vi "Format Control Data Element.vi"(6 "Unsupported Error":errorcluster, 8 "error in (no error)":errorcluster, 10 "Content Type in":string, 11 "Data":variant) -> (0 "error out":errorcluster, 2 "Content Type out":string, 3 "JSON string":string)   [LabVIEW 2023, in "Response.lvclass"]
uses:
  Response.lvclass
  <vilib>/Utility/Data Type/Type Definitions/Data Type.ctl
  Helpers/UTC.ctl
  <vilib>/Utility/Data Type/NI_Data Type.lvlib
  <vilib>/wsapi/NI_WebServices.lvlib
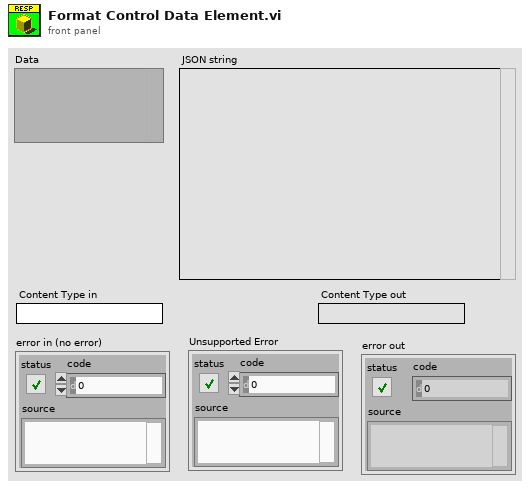
[diagram p1: front panel]
types:
  T1 = typedef "NI_Data Type.lvlib/Data Type.ctl" = enum8{"Invalid Type", "Void", "I8", "I16", "I32", "I64", "U8", "U16", "U32", "U64", "Single Float", "Double Float", "Extended Float", "Single Complex", "Double Complex", "Extended Complex", "Enum U8", "Enum U16", "Enum U32", "Enum U64", "Single Float With Unit", "Double Float With Unit", "Extended Float With Unit", "Single Complex with Unit", "Double Complex with Unit", "Extended Complex with Unit", "Boolean", "String", "Path", "Picture", "Tag", "Array", "Cluster", "Variant", "LV Variant", "Waveform", "Timestamp", "Digital Waveform", "Digital Data", "ExpressData", "Refnum", "External Data", "VI", "Poly VI", "LabVIEW Class Instance", "Fixed Point", "Set Collection", "Map Collection"}
  T2 = typedef "NI_Data Type.lvlib/Type Definition Info.ctl" = cluster{"Name":string, "Timestamp":u32}
  T3 = typedef "UTC.ctl" = string
  T4 = cluster{"t0":timestamp, "Y":dbl[], "dt":dbl, "attributes":variant}
  T5 = cluster{"t0":timestamp, "dt":dbl, "attributes":variant, "Y":digitaldata}
  T6 = typedef "imagedata.ctl" = cluster{"image type":i32, "image depth":i32, "image":u8[], "mask":u8[], "colors":u32[], "Rectangle":cluster{"left":i16, "top":i16, "right":i16, "bottom":i16}}
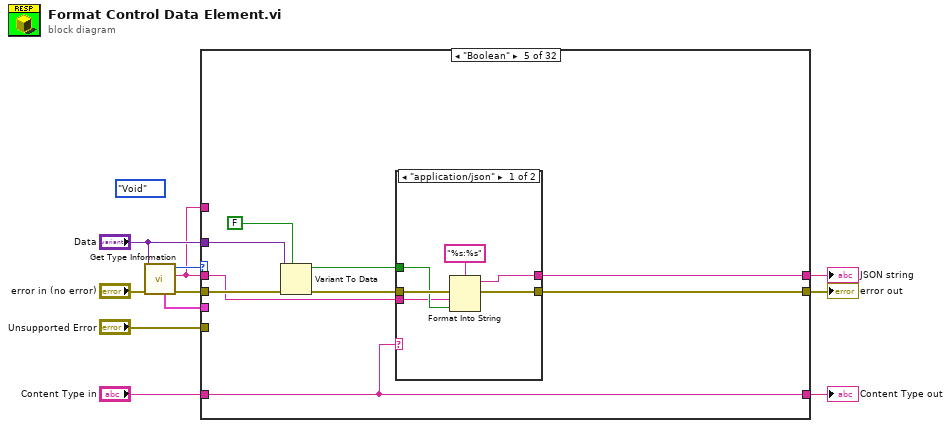
[diagram p0: block diagram]
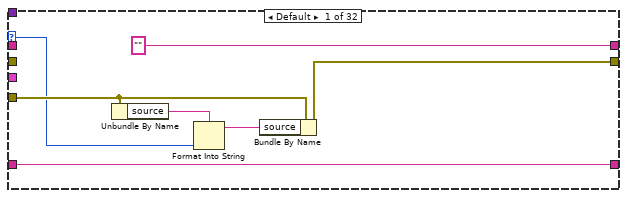
[diagram p2: hidden frame]
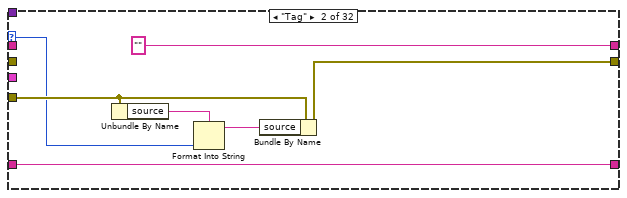
[diagram p3: hidden frame]
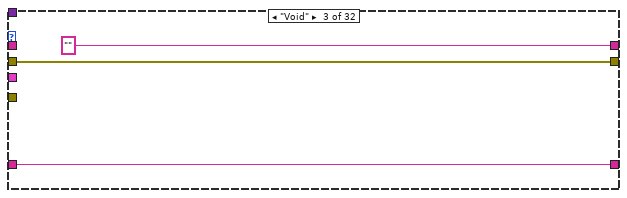
[diagram p4: hidden frame]
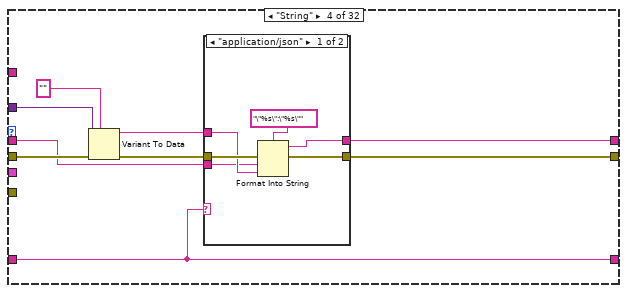
[diagram p5: hidden frame]
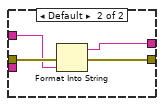
[diagram p6: hidden frame]
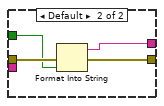
[diagram p7: hidden frame]
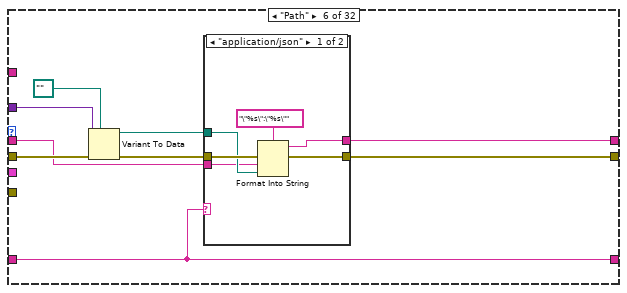
[diagram p8: hidden frame]
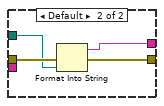
[diagram p9: hidden frame]
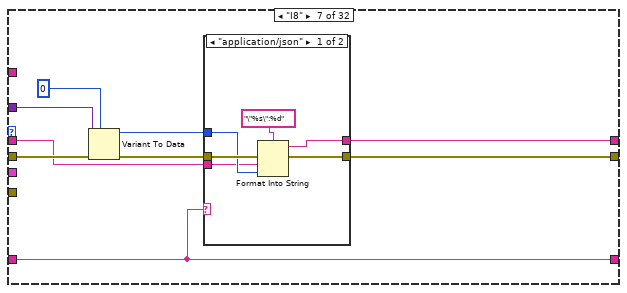
[diagram p10: hidden frame]
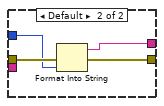
[diagram p11: hidden frame]
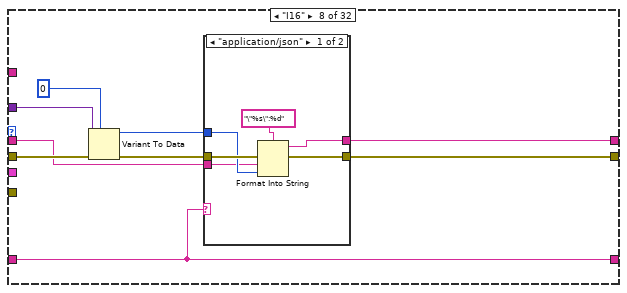
[diagram p12: hidden frame]
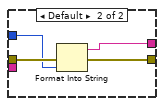
[diagram p13: hidden frame]
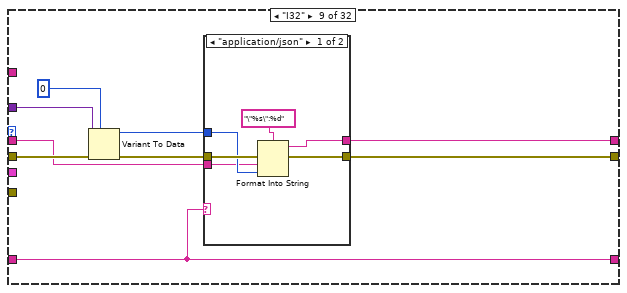
[diagram p14: hidden frame]
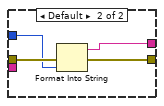
[diagram p15: hidden frame]
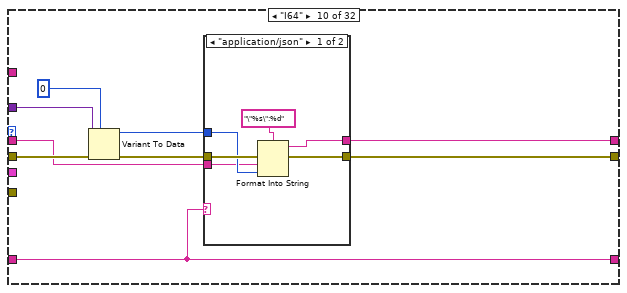
[diagram p16: hidden frame]
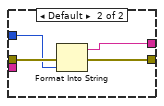
[diagram p17: hidden frame]
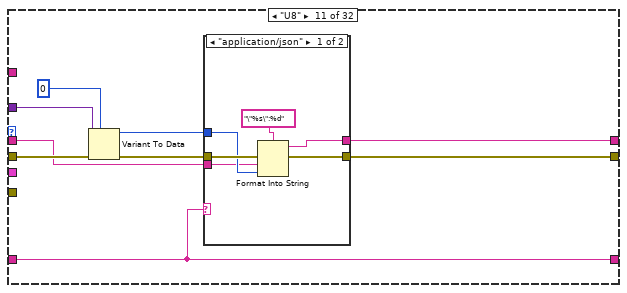
[diagram p18: hidden frame]
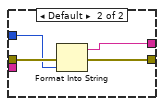
[diagram p19: hidden frame]
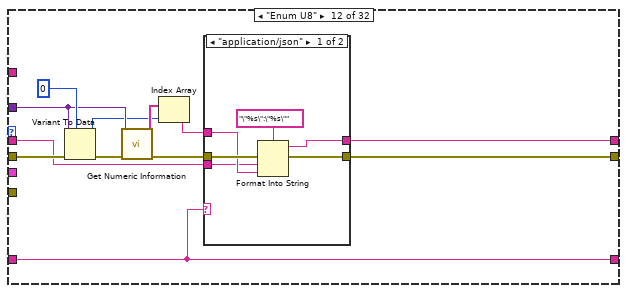
[diagram p20: hidden frame]
diagram:
  (unwired) Data_Type."Void" ("type")
  n1 = call <vilib>:"Get Type Information.vi"("error in (no error)"="error in (no error)", "variant"="Data") -> ("error out"=w7:errorcluster, "name"=w1:string, "type"=w8:T1, "type definition info"=w9:T2)  [unwired: 5 in, 1 out]
  n2 = case shown="\"Boolean\"" w8 {
    selector: w8 -> [w12 w19 _ _ _ _ _ _ _ _ _ _ _ _ _ _ _ _ _ _ _ _ _ _ _ _ _ _ _ _ _ _]
    tunnel: w7 -> [_ _ w28 w37 w56 w75 w94 w113 w132 w151 w170 w192 w214 w236 w258 w277 w296 w315 w334 w353 w372 w391 w410 w429 w449 w478 w494 w505 w514 w528 w1329 w1344]
    tunnel: w9 -> [_ _ _ _ _ _ _ _ _ _ _ _ _ _ _ _ _ _ _ _ _ _ _ _ _ _ _ _ _ _ _ _]
    tunnel: [w15 w22 w28 w34 w53 w72 w91 w110 w129 w148 w167 w191 w213 w235 w257 w274 w293 w312 w331 w350 w369 w388 w407 w426 w446 w474 w491 w502 w508 w530 w1320 w1352] -> w4
    tunnel: ["" "" "" w32 w51 w70 w89 w108 w127 w146 w165 w190 w212 w234 w256 w272 w291 w310 w329 w348 w367 w386 w405 w424 w444 w470 w487 w498 w506 w519 w1319 w1351] -> w3
    tunnel: "Data" -> [_ _ _ w36 w55 w74 w93 w112 w131 w150 w169 w185 w207 w229 w251 w276 w295 w314 w333 w352 w371 w390 w409 w428 w448 w477 w493 w504 w513 w527 w1328 w1346]
    tunnel: "Content Type in" -> [w18 w25 w26 w30 w49 w68 w87 w106 w125 w144 w163 w188 w210 w232 w254 w270 w289 w308 w327 w346 w365 w384 w403 w422 w442 w471 w488 w499 _ _ _ _]
    tunnel: [w18 w25 w26 w30 w49 w68 w87 w106 w125 w144 w163 w188 w210 w232 w254 w270 w289 w308 w327 w346 w365 w384 w403 w422 w442 w472 w489 w500 "image/png" "application/json" w1318 w1350] -> w2
    tunnel: "Unsupported Error" -> [w16 w23 _ _ _ _ _ _ _ _ _ _ _ _ _ _ _ _ _ _ _ _ _ _ _ w473 w490 w501 _ w521 w1325 w1357]
    tunnel: w1 -> [_ _ _ w29 w48 w67 w86 w105 w124 w143 w162 w187 w209 w231 w253 w269 w288 w307 w326 w345 w364 w383 w402 w421 w441 _ _ _ _ _ _ _]
    tunnel: w1 -> [_ _ _ _ _ _ _ _ _ _ _ _ _ _ _ _ _ _ _ _ _ _ _ _ _ _ _ _ _ w516 w1315 _]
    frame Default {
      n3 = Unbundle By Name(w16) -> ("source"=w14:string)
      n4 = Format Into String(format string=w14, w12) -> (resulting string=w13:string)  [unwired: 2 in, 1 out]
      n5 = Bundle By Name(cluster=w16, "source"=w13) -> (w15:errorcluster)
    }
    frame "Tag" {
      n6 = Unbundle By Name(w23) -> ("source"=w21:string)
      n7 = Format Into String(format string=w21, w19) -> (resulting string=w20:string)  [unwired: 2 in, 1 out]
      n8 = Bundle By Name(cluster=w23, "source"=w20) -> (w22:errorcluster)
    }
    frame "Void" {
    }
    frame "String" {
      n9 = Variant To Data(error in=w37, type="", Variant=w36) -> (data=w33:string, error out=w35:errorcluster)
      n10 = case shown="\"application/json\"" w30 {
        tunnel: w35 -> [w43 w47]
        tunnel: [w42 w46] -> w34
        tunnel: w33 -> [w39 w45]
        tunnel: [w40 w44] -> w32
        tunnel: w29 -> [w38 _]
        frame "application/json" {
          n11 = Format Into String(format string="\"%s\":\"%s\"", error in=w43, w38, w39) -> (resulting string=w40:string, error out=w42:errorcluster)  [unwired: 1 in]
        }
        frame Default {
          n12 = Format Into String(error in=w47, w45) -> (resulting string=w44:string, error out=w46:errorcluster)  [unwired: 2 in]
        }
      }
    }
    frame "Boolean" {
      n13 = Variant To Data(error in=w56, type=FALSE, Variant=w55) -> (data=w52:bool, error out=w54:errorcluster)
      n14 = case shown="\"application/json\"" w49 {
        tunnel: w54 -> [w62 w66]
        tunnel: [w61 w65] -> w53
        tunnel: w52 -> [w58 w64]
        tunnel: [w59 w63] -> w51
        tunnel: w48 -> [w57 _]
        frame "application/json" {
          n15 = Format Into String(format string="%s:%s", error in=w62, w57, w58) -> (resulting string=w59:string, error out=w61:errorcluster)  [unwired: 1 in]
        }
        frame Default {
          n16 = Format Into String(error in=w66, w64) -> (resulting string=w63:string, error out=w65:errorcluster)  [unwired: 2 in]
        }
      }
    }
    frame "Path" {
      n17 = Variant To Data(error in=w75, type=path "", Variant=w74) -> (data=w71:path, error out=w73:errorcluster)
      n18 = case shown="\"application/json\"" w68 {
        tunnel: w73 -> [w81 w85]
        tunnel: [w80 w84] -> w72
        tunnel: w71 -> [w79 w83]
        tunnel: [w77 w82] -> w70
        tunnel: w67 -> [w76 _]
        frame "application/json" {
          n19 = Format Into String(format string="\"%s\":\"%s\"", error in=w81, w76, w79) -> (resulting string=w77:string, error out=w80:errorcluster)  [unwired: 1 in]
        }
        frame Default {
          n20 = Format Into String(error in=w85, w83) -> (resulting string=w82:string, error out=w84:errorcluster)  [unwired: 2 in]
        }
      }
    }
    frame "I8" {
      n21 = Variant To Data(error in=w94, type=i8 0, Variant=w93) -> (data=w90:i8, error out=w92:errorcluster)
      n22 = case shown="\"application/json\"" w87 {
        tunnel: w92 -> [w100 w104]
        tunnel: [w99 w103] -> w91
        tunnel: w90 -> [w98 w102]
        tunnel: [w96 w101] -> w89
        tunnel: w86 -> [w95 _]
        frame "application/json" {
          n23 = Format Into String(format string="\"%s\":%d", error in=w100, w95, w98) -> (resulting string=w96:string, error out=w99:errorcluster)  [unwired: 1 in]
        }
        frame Default {
          n24 = Format Into String(error in=w104, w102) -> (resulting string=w101:string, error out=w103:errorcluster)  [unwired: 2 in]
        }
      }
    }
    frame "I16" {
      n25 = Variant To Data(error in=w113, type=i16 0, Variant=w112) -> (data=w109:i16, error out=w111:errorcluster)
      n26 = case shown="\"application/json\"" w106 {
        tunnel: w111 -> [w119 w123]
        tunnel: [w118 w122] -> w110
        tunnel: w109 -> [w117 w121]
        tunnel: [w115 w120] -> w108
        tunnel: w105 -> [w114 _]
        frame "application/json" {
          n27 = Format Into String(format string="\"%s\":%d", error in=w119, w114, w117) -> (resulting string=w115:string, error out=w118:errorcluster)  [unwired: 1 in]
        }
        frame Default {
          n28 = Format Into String(error in=w123, w121) -> (resulting string=w120:string, error out=w122:errorcluster)  [unwired: 2 in]
        }
      }
    }
    frame "I32" {
      n29 = Variant To Data(error in=w132, type=0, Variant=w131) -> (data=w128:i32, error out=w130:errorcluster)
      n30 = case shown="\"application/json\"" w125 {
        tunnel: w130 -> [w138 w142]
        tunnel: [w137 w141] -> w129
        tunnel: w128 -> [w136 w140]
        tunnel: [w134 w139] -> w127
        tunnel: w124 -> [w133 _]
        frame "application/json" {
          n31 = Format Into String(format string="\"%s\":%d", error in=w138, w133, w136) -> (resulting string=w134:string, error out=w137:errorcluster)  [unwired: 1 in]
        }
        frame Default {
          n32 = Format Into String(error in=w142, w140) -> (resulting string=w139:string, error out=w141:errorcluster)  [unwired: 2 in]
        }
      }
    }
    frame "I64" {
      n33 = Variant To Data(error in=w151, type=i64 0, Variant=w150) -> (data=w147:i64, error out=w149:errorcluster)
      n34 = case shown="\"application/json\"" w144 {
        tunnel: w149 -> [w157 w161]
        tunnel: [w156 w160] -> w148
        tunnel: w147 -> [w155 w159]
        tunnel: [w153 w158] -> w146
        tunnel: w143 -> [w152 _]
        frame "application/json" {
          n35 = Format Into String(format string="\"%s\":%d", error in=w157, w152, w155) -> (resulting string=w153:string, error out=w156:errorcluster)  [unwired: 1 in]
        }
        frame Default {
          n36 = Format Into String(error in=w161, w159) -> (resulting string=w158:string, error out=w160:errorcluster)  [unwired: 2 in]
        }
      }
    }
    frame "U8" {
      n37 = Variant To Data(error in=w170, type=u8 0, Variant=w169) -> (data=w166:u8, error out=w168:errorcluster)
      n38 = case shown="\"application/json\"" w163 {
        tunnel: w168 -> [w176 w180]
        tunnel: [w175 w179] -> w167
        tunnel: w166 -> [w174 w178]
        tunnel: [w172 w177] -> w165
        tunnel: w162 -> [w171 _]
        frame "application/json" {
          n39 = Format Into String(format string="\"%s\":%d", error in=w176, w171, w174) -> (resulting string=w172:string, error out=w175:errorcluster)  [unwired: 1 in]
        }
        frame Default {
          n40 = Format Into String(error in=w180, w178) -> (resulting string=w177:string, error out=w179:errorcluster)  [unwired: 2 in]
        }
      }
    }
    frame "Enum U8" {
      n41 = Variant To Data(error in=w192, type=u8 0, Variant=w185) -> (data=w184:u8, error out=w183:errorcluster)
      n42 = call <vilib>:"Get Numeric Information.vi"("error in (no error)"=w183, "variant"=w185) -> ("error out"=w181:errorcluster, "enum names"=w186:string[])  [unwired: 6 in, 2 out]
      n43 = Index Array(array=w186, index=w184) -> (element=w182:string)
      n44 = case shown="\"application/json\"" w188 {
        tunnel: w181 -> [w198 w202]
        tunnel: [w197 w201] -> w191
        tunnel: w182 -> [w196 w200]
        tunnel: [w194 w199] -> w190
        tunnel: w187 -> [w193 _]
        frame "application/json" {
          n45 = Format Into String(format string="\"%s\":\"%s\"", error in=w198, w193, w196) -> (resulting string=w194:string, error out=w197:errorcluster)  [unwired: 1 in]
        }
        frame Default {
          n46 = Format Into String(error in=w202, w200) -> (resulting string=w199:string, error out=w201:errorcluster)  [unwired: 2 in]
        }
      }
    }
    frame "Enum U16" {
      n47 = Variant To Data(error in=w214, type=u16 0, Variant=w207) -> (data=w206:u16, error out=w205:errorcluster)
      n48 = call <vilib>:"Get Numeric Information.vi"("error in (no error)"=w205, "variant"=w207) -> ("error out"=w203:errorcluster, "enum names"=w208:string[])  [unwired: 6 in, 2 out]
      n49 = Index Array(array=w208, index=w206) -> (element=w204:string)
      n50 = case shown="\"application/json\"" w210 {
        tunnel: w203 -> [w220 w224]
        tunnel: [w219 w223] -> w213
        tunnel: w204 -> [w218 w222]
        tunnel: [w216 w221] -> w212
        tunnel: w209 -> [w215 _]
        frame "application/json" {
          n51 = Format Into String(format string="\"%s\":\"%s\"", error in=w220, w215, w218) -> (resulting string=w216:string, error out=w219:errorcluster)  [unwired: 1 in]
        }
        frame Default {
          n52 = Format Into String(error in=w224, w222) -> (resulting string=w221:string, error out=w223:errorcluster)  [unwired: 2 in]
        }
      }
    }
    frame "Enum U32" {
      n53 = Variant To Data(error in=w236, type=u32 0, Variant=w229) -> (data=w228:u32, error out=w227:errorcluster)
      n54 = call <vilib>:"Get Numeric Information.vi"("error in (no error)"=w227, "variant"=w229) -> ("error out"=w225:errorcluster, "enum names"=w230:string[])  [unwired: 6 in, 2 out]
      n55 = Index Array(array=w230, index=w228) -> (element=w226:string)
      n56 = case shown="\"application/json\"" w232 {
        tunnel: w225 -> [w242 w246]
        tunnel: [w241 w245] -> w235
        tunnel: w226 -> [w240 w244]
        tunnel: [w238 w243] -> w234
        tunnel: w231 -> [w237 _]
        frame "application/json" {
          n57 = Format Into String(format string="\"%s\":\"%s\"", error in=w242, w237, w240) -> (resulting string=w238:string, error out=w241:errorcluster)  [unwired: 1 in]
        }
        frame Default {
          n58 = Format Into String(error in=w246, w244) -> (resulting string=w243:string, error out=w245:errorcluster)  [unwired: 2 in]
        }
      }
    }
    frame "Enum U64" {
      n59 = Variant To Data(error in=w258, type=u64 0, Variant=w251) -> (data=w250:u64, error out=w249:errorcluster)
      n60 = call <vilib>:"Get Numeric Information.vi"("error in (no error)"=w249, "variant"=w251) -> ("error out"=w247:errorcluster, "enum names"=w252:string[])  [unwired: 6 in, 2 out]
      n61 = Index Array(array=w252, index=w250) -> (element=w248:string)
      n62 = case shown="\"application/json\"" w254 {
        tunnel: w247 -> [w264 w268]
        tunnel: [w263 w267] -> w257
        tunnel: w248 -> [w262 w266]
        tunnel: [w260 w265] -> w256
        tunnel: w253 -> [w259 _]
        frame "application/json" {
          n63 = Format Into String(format string="\"%s\":\"%s\"", error in=w264, w259, w262) -> (resulting string=w260:string, error out=w263:errorcluster)  [unwired: 1 in]
        }
        frame Default {
          n64 = Format Into String(error in=w268, w266) -> (resulting string=w265:string, error out=w267:errorcluster)  [unwired: 2 in]
        }
      }
    }
    frame "U16" {
      n65 = Variant To Data(error in=w277, type=u16 0, Variant=w276) -> (data=w273:u16, error out=w275:errorcluster)
      n66 = case shown="\"application/json\"" w270 {
        tunnel: w275 -> [w283 w287]
        tunnel: [w282 w286] -> w274
        tunnel: w273 -> [w281 w285]
        tunnel: [w279 w284] -> w272
        tunnel: w269 -> [w278 _]
        frame "application/json" {
          n67 = Format Into String(format string="\"%s\":%d", error in=w283, w278, w281) -> (resulting string=w279:string, error out=w282:errorcluster)  [unwired: 1 in]
        }
        frame Default {
          n68 = Format Into String(error in=w287, w285) -> (resulting string=w284:string, error out=w286:errorcluster)  [unwired: 2 in]
        }
      }
    }
    frame "U32" {
      n69 = Variant To Data(error in=w296, type=u32 0, Variant=w295) -> (data=w292:u32, error out=w294:errorcluster)
      n70 = case shown="\"application/json\"" w289 {
        tunnel: w294 -> [w302 w306]
        tunnel: [w301 w305] -> w293
        tunnel: w292 -> [w300 w304]
        tunnel: [w298 w303] -> w291
        tunnel: w288 -> [w297 _]
        frame "application/json" {
          n71 = Format Into String(format string="\"%s\":%d", error in=w302, w297, w300) -> (resulting string=w298:string, error out=w301:errorcluster)  [unwired: 1 in]
        }
        frame Default {
          n72 = Format Into String(error in=w306, w304) -> (resulting string=w303:string, error out=w305:errorcluster)  [unwired: 2 in]
        }
      }
    }
    frame "U64" {
      n73 = Variant To Data(error in=w315, type=u64 0, Variant=w314) -> (data=w311:u64, error out=w313:errorcluster)
      n74 = case shown="\"application/json\"" w308 {
        tunnel: w313 -> [w321 w325]
        tunnel: [w320 w324] -> w312
        tunnel: w311 -> [w319 w323]
        tunnel: [w317 w322] -> w310
        tunnel: w307 -> [w316 _]
        frame "application/json" {
          n75 = Format Into String(format string="\"%s\":%d", error in=w321, w316, w319) -> (resulting string=w317:string, error out=w320:errorcluster)  [unwired: 1 in]
        }
        frame Default {
          n76 = Format Into String(error in=w325, w323) -> (resulting string=w322:string, error out=w324:errorcluster)  [unwired: 2 in]
        }
      }
    }
    frame "Single Float" {
      n77 = Variant To Data(error in=w334, type=sgl 0.0, Variant=w333) -> (data=w330:sgl, error out=w332:errorcluster)
      n78 = case shown="\"application/json\"" w327 {
        tunnel: w332 -> [w340 w344]
        tunnel: [w339 w343] -> w331
        tunnel: w330 -> [w338 w342]
        tunnel: [w336 w341] -> w329
        tunnel: w326 -> [w335 _]
        frame "application/json" {
          n79 = Format Into String(format string="\"%s\":%f", error in=w340, w335, w338) -> (resulting string=w336:string, error out=w339:errorcluster)  [unwired: 1 in]
        }
        frame Default {
          n80 = Format Into String(error in=w344, w342) -> (resulting string=w341:string, error out=w343:errorcluster)  [unwired: 2 in]
        }
      }
    }
    frame "Double Float" {
      n81 = Variant To Data(error in=w353, type=0.0, Variant=w352) -> (data=w349:dbl, error out=w351:errorcluster)
      n82 = case shown="\"application/json\"" w346 {
        tunnel: w351 -> [w359 w363]
        tunnel: [w358 w362] -> w350
        tunnel: w349 -> [w357 w361]
        tunnel: [w355 w360] -> w348
        tunnel: w345 -> [w354 _]
        frame "application/json" {
          n83 = Format Into String(format string="\"%s\":%f", error in=w359, w354, w357) -> (resulting string=w355:string, error out=w358:errorcluster)  [unwired: 1 in]
        }
        frame Default {
          n84 = Format Into String(error in=w363, w361) -> (resulting string=w360:string, error out=w362:errorcluster)  [unwired: 2 in]
        }
      }
    }
    frame "Extended Float" {
      n85 = Variant To Data(error in=w372, type=ext 0.0, Variant=w371) -> (data=w368:ext, error out=w370:errorcluster)
      n86 = case shown="\"application/json\"" w365 {
        tunnel: w370 -> [w378 w382]
        tunnel: [w377 w381] -> w369
        tunnel: w368 -> [w376 w380]
        tunnel: [w374 w379] -> w367
        tunnel: w364 -> [w373 _]
        frame "application/json" {
          n87 = Format Into String(format string="\"%s\":%f", error in=w378, w373, w376) -> (resulting string=w374:string, error out=w377:errorcluster)  [unwired: 1 in]
        }
        frame Default {
          n88 = Format Into String(error in=w382, w380) -> (resulting string=w379:string, error out=w381:errorcluster)  [unwired: 2 in]
        }
      }
    }
    frame "Single Complex" {
      n89 = Variant To Data(error in=w391, type=csg 0.0+0.0i, Variant=w390) -> (data=w387:csg, error out=w389:errorcluster)
      n90 = case shown="\"application/json\"" w384 {
        tunnel: w389 -> [w397 w401]
        tunnel: [w396 w400] -> w388
        tunnel: w387 -> [w395 w399]
        tunnel: [w393 w398] -> w386
        tunnel: w383 -> [w392 _]
        frame "application/json" {
          n91 = Format Into String(format string="\"%s\":%f", error in=w397, w392, w395) -> (resulting string=w393:string, error out=w396:errorcluster)  [unwired: 1 in]
        }
        frame Default {
          n92 = Format Into String(error in=w401, w399) -> (resulting string=w398:string, error out=w400:errorcluster)  [unwired: 2 in]
        }
      }
    }
    frame "Double Complex" {
      n93 = Variant To Data(error in=w410, type=cdb 0.0+0.0i, Variant=w409) -> (data=w406:cdb, error out=w408:errorcluster)
      n94 = case shown="\"application/json\"" w403 {
        tunnel: w408 -> [w416 w420]
        tunnel: [w415 w419] -> w407
        tunnel: w406 -> [w414 w418]
        tunnel: [w412 w417] -> w405
        tunnel: w402 -> [w411 _]
        frame "application/json" {
          n95 = Format Into String(format string="\"%s\":%f", error in=w416, w411, w414) -> (resulting string=w412:string, error out=w415:errorcluster)  [unwired: 1 in]
        }
        frame Default {
          n96 = Format Into String(error in=w420, w418) -> (resulting string=w417:string, error out=w419:errorcluster)  [unwired: 2 in]
        }
      }
    }
    frame "Extended Complex" {
      n97 = Variant To Data(error in=w429, type=cxt 0.0+0.0i, Variant=w428) -> (data=w425:cxt, error out=w427:errorcluster)
      n98 = case shown="\"application/json\"" w422 {
        tunnel: w427 -> [w435 w439]
        tunnel: [w434 w438] -> w426
        tunnel: w425 -> [w433 w437]
        tunnel: [w431 w436] -> w424
        tunnel: w421 -> [w430 _]
        frame "application/json" {
          n99 = Format Into String(format string="\"%s\":%f", error in=w435, w430, w433) -> (resulting string=w431:string, error out=w434:errorcluster)  [unwired: 1 in]
        }
        frame Default {
          n100 = Format Into String(error in=w439, w437) -> (resulting string=w436:string, error out=w438:errorcluster)  [unwired: 2 in]
        }
      }
    }
    frame "Timestamp" {
      n101 = Variant To Data(error in=w449, type=timestamp(0 s since 1904-01-01), Variant=w448) -> (data=w445:timestamp, error out=w447:errorcluster)
      n102 = case shown="\"application/json\"" w442 {
        tunnel: w447 -> [w457 w462]
        tunnel: [w456 w461] -> w446
        tunnel: w445 -> [w451 w460]
        tunnel: [w454 w459] -> w444
        tunnel: w441 -> [w453 _]
        tunnel: T3 "%^<%Y-%m-%dT%H:%M:%S%3u>TZ" ("UTC") -> [w452 w458]
        frame "application/json" {
          n103 = Format Into String(format string=w452, w451) -> (resulting string=w450:string)  [unwired: 2 in, 1 out]
          n104 = Format Into String(format string="\"%s\":\"%s\"", error in=w457, w453, w450) -> (resulting string=w454:string, error out=w456:errorcluster)  [unwired: 1 in]
        }
        frame Default {
          n105 = Format Into String(format string=w458, error in=w462, w460) -> (resulting string=w459:string, error out=w461:errorcluster)  [unwired: 1 in]
        }
      }
    }
    frame "Waveform" {
      # "#TODO: Make this work"
      n106 = Variant To Data(error in=w478, type=waveform(dbl) {"t0"=timestamp(0 s since 1904-01-01), "dt"=1.0, "Y"=[]}, Variant=w477) -> (data=w469:waveform(dbl), error out=w475:errorcluster)
      n107 = Unbundle By Name(w469) -> ("t0"=w467:timestamp, "dt"=w466:dbl, "Y"=w465:dbl[], "attributes"=w464:variant)
      n108 = Bundle By Name(cluster=T4 {"t0"=timestamp(0 s since 1904-01-01), "Y"=[], "dt"=1.0, "attributes"=variant}, "t0"=w467, "dt"=w466, "Y"=w465, "attributes"=w464) -> (w463:T4)
      n109 = call "Format Control Data Element.vi"("Unsupported Error"=w473, "error in (no error)"=w475, "Content Type in"=w471, "Data"=w463) -> ("error out"=w474:errorcluster, "Content Type out"=w472:string, "JSON string"=w470:string)  [unwired: 5 in]
    }
    frame "Digital Waveform" {
      # "#TODO: Make this work"
      n110 = call <vilib>:"DWDT Empty Digital.vi"() -> ("digital waveform out"=w480:digitalwaveform)  [unwired: 5 in]
      n111 = Variant To Data(error in=w494, type=w480, Variant=w493) -> (data=w486:digitalwaveform, error out=w492:errorcluster)
      n112 = Unbundle By Name(w486) -> ("t0"=w484:timestamp, "dt"=w483:dbl, "Y"=w479:digitaldata, "attributes"=w482:variant)
      n113 = Bundle By Name(cluster=T5 {"t0"=timestamp(0 s since 1904-01-01), "dt"=1.0, "attributes"=variant, "Y"={"transitions"=[], "data"=[]}}, "t0"=w484, "dt"=w483, "Y"=w479, "attributes"=w482) -> (w481:T5)
      n114 = call "Format Control Data Element.vi"("Unsupported Error"=w490, "error in (no error)"=w492, "Content Type in"=w488, "Data"=w481) -> ("error out"=w491:errorcluster, "Content Type out"=w489:string, "JSON string"=w487:string)  [unwired: 5 in]
    }
    frame "Digital Data" {
      # "#TODO: Make this work"
      n115 = call <vilib>:"DTbl Empty Digital.vi"() -> ("digital data"=w497:digitaldata)  [unwired: 5 in]
      n116 = Variant To Data(error in=w505, type=w497, Variant=w504) -> (data=w496:digitaldata, error out=w503:errorcluster)
      n117 = Unbundle By Name(w496) -> ("data"=w495:u8[][])
      n118 = call "Format Control Data Element.vi"("Unsupported Error"=w501, "error in (no error)"=w503, "Content Type in"=w499, "Data"=w495) -> ("error out"=w502:errorcluster, "Content Type out"=w500:string, "JSON string"=w498:string)  [unwired: 5 in]
    }
    frame "Picture" {
      # "#TODO: Make this work"
      n119 = call "Empty Picture"() -> ("empty picture"=w512:picture)
      n120 = Variant To Data(error in=w514, type=w512, Variant=w513) -> (data=w510:picture, error out=w509:errorcluster)
      n121 = call <vilib>:"Picture to Pixmap.vi"("picture"=w510) -> ("image data"=w507:T6)  [unwired: 9 in, 1 out]
      n122 = call <vilib>:"LV Image to PNG Data.vi"("error in (no error)"=w509, "image data"=w507) -> ("error out"=w508:errorcluster, "png data"=w506:string)  [unwired: 8 in]
    }
    frame "Array" {
      # "#TODO: Make this work"
      n123 = call <vilib>:"Get Array Information.vi"("error in (no error)"=w528, "variant"=w527) -> ("error out"=w526:errorcluster, "array element data type"=w525:variant, "number of dimensions"=w522:i32)  [unwired: 6 in, 1 out]
      n124 = call <vilib>:"Get Type Information.vi"("error in (no error)"=w526, "variant"=w525) -> ("error out"=w524:errorcluster, "type"=w523:T1)  [unwired: 5 in, 3 out]
      n125 = case shown="\"Enum U32\"" w523 {
        tunnel: ["" ("JSON string") w538 w578 w618 w658 w698 w738 w778 w818 w858 w898 w938 w978 w1018 w1058 w1098 w1138 w1178 w1199 w1224 w1248 w1272 w1296] -> w520
        tunnel: [w532 w537 w577 w617 w657 w697 w737 w777 w817 w857 w897 w937 w977 w1017 w1057 w1097 w1137 w1177 w1198 w1223 w1247 w1271 w1295] -> w530
        tunnel: w527 -> [_ w536 w576 w616 w656 w696 w736 w776 w816 w856 w896 w936 w976 w1016 w1056 w1096 w1136 w1176 w1197 w1222 w1246 w1270 w1294]
        tunnel: w524 -> [w532 w535 w575 w615 w655 w695 w735 w775 w815 w855 w895 w935 w975 w1015 w1055 w1095 w1135 w1175 w1196 w1221 w1245 w1269 w1293]
        tunnel: w522 -> [_ w534 w574 w614 w654 w694 w734 w774 w814 w854 w894 w934 w974 w1014 w1054 w1094 w1134 w1174 w1195 w1220 w1244 w1268 w1292]
        tunnel: w521 -> [_ _ _ _ _ _ _ _ _ _ _ _ _ _ _ _ _ _ _ w1218 w1242 w1266 w1290]
        frame Default {
        }
        frame "I8" {
          n126 = case shown="0, Default" w534 {
            tunnel: ["" ("JSON string") w547 w555 w563 w571] -> w538
            tunnel: [w540 w546 w554 w562 w570] -> w537
            tunnel: w536 -> [_ w545 w553 w561 w569]
            tunnel: w535 -> [w540 w544 w552 w560 w568]
            tunnel: i8 0 -> [_ w542 w550 w558 w566]
            frame 0, Default {
            }
            frame 1 {
              n127 = Initialize Array(w542) -> (w541:i8[])  [unwired: 1 in]
              n128 = Variant To Data(error in=w544, type=w541, Variant=w545) -> (data=w543:i8[], error out=w548:errorcluster)
              n129 = Flatten To JSON(anything=w543, error in (no error)=w548) -> (JSON string=w547:string, 11:w546:errorcluster)  [unwired: 1 in]
            }
            frame 2 {
              n130 = Initialize Array(w550) -> (w549:i8[][])  [unwired: 2 in]
              n131 = Variant To Data(error in=w552, type=w549, Variant=w553) -> (data=w551:i8[][], error out=w556:errorcluster)
              n132 = Flatten To JSON(anything=w551, error in (no error)=w556) -> (JSON string=w555:string, 11:w554:errorcluster)  [unwired: 1 in]
            }
            frame 3 {
              n133 = Initialize Array(w558) -> (w557:i8[][][])  [unwired: 3 in]
              n134 = Variant To Data(error in=w560, type=w557, Variant=w561) -> (data=w559:i8[][][], error out=w564:errorcluster)
              n135 = Flatten To JSON(anything=w559, error in (no error)=w564) -> (JSON string=w563:string, 11:w562:errorcluster)  [unwired: 1 in]
            }
            frame 4 {
              n136 = Initialize Array(w566) -> (w565:i8[][][][])  [unwired: 4 in]
              n137 = Variant To Data(error in=w568, type=w565, Variant=w569) -> (data=w567:i8[][][][], error out=w572:errorcluster)
              n138 = Flatten To JSON(anything=w567, error in (no error)=w572) -> (JSON string=w571:string, 11:w570:errorcluster)  [unwired: 1 in]
            }
          }
        }
        frame "I16" {
          n139 = case shown="1" w574 {
            tunnel: ["" ("JSON string") w587 w595 w603 w611] -> w578
            tunnel: [w580 w586 w594 w602 w610] -> w577
            tunnel: w576 -> [_ w585 w593 w601 w609]
            tunnel: w575 -> [w580 w584 w592 w600 w608]
            tunnel: i16 0 -> [_ w582 w590 w598 w606]
            frame 0, Default {
            }
            frame 1 {
              n140 = Initialize Array(w582) -> (w581:i16[])  [unwired: 1 in]
              n141 = Variant To Data(error in=w584, type=w581, Variant=w585) -> (data=w583:i16[], error out=w588:errorcluster)
              n142 = Flatten To JSON(anything=w583, error in (no error)=w588) -> (JSON string=w587:string, 11:w586:errorcluster)  [unwired: 1 in]
            }
            frame 2 {
              n143 = Initialize Array(w590) -> (w589:i16[][])  [unwired: 2 in]
              n144 = Variant To Data(error in=w592, type=w589, Variant=w593) -> (data=w591:i16[][], error out=w596:errorcluster)
              n145 = Flatten To JSON(anything=w591, error in (no error)=w596) -> (JSON string=w595:string, 11:w594:errorcluster)  [unwired: 1 in]
            }
            frame 3 {
              n146 = Initialize Array(w598) -> (w597:i16[][][])  [unwired: 3 in]
              n147 = Variant To Data(error in=w600, type=w597, Variant=w601) -> (data=w599:i16[][][], error out=w604:errorcluster)
              n148 = Flatten To JSON(anything=w599, error in (no error)=w604) -> (JSON string=w603:string, 11:w602:errorcluster)  [unwired: 1 in]
            }
            frame 4 {
              n149 = Initialize Array(w606) -> (w605:i16[][][][])  [unwired: 4 in]
              n150 = Variant To Data(error in=w608, type=w605, Variant=w609) -> (data=w607:i16[][][][], error out=w612:errorcluster)
              n151 = Flatten To JSON(anything=w607, error in (no error)=w612) -> (JSON string=w611:string, 11:w610:errorcluster)  [unwired: 1 in]
            }
          }
        }
        frame "I32" {
          n152 = case shown="1" w614 {
            tunnel: ["" ("JSON string") w627 w635 w643 w651] -> w618
            tunnel: [w620 w626 w634 w642 w650] -> w617
            tunnel: w616 -> [_ w625 w633 w641 w649]
            tunnel: w615 -> [w620 w624 w632 w640 w648]
            tunnel: 0 -> [_ w622 w630 w638 w646]
            frame 0, Default {
            }
            frame 1 {
              n153 = Initialize Array(w622) -> (w621:i32[])  [unwired: 1 in]
              n154 = Variant To Data(error in=w624, type=w621, Variant=w625) -> (data=w623:i32[], error out=w628:errorcluster)
              n155 = Flatten To JSON(anything=w623, error in (no error)=w628) -> (JSON string=w627:string, 11:w626:errorcluster)  [unwired: 1 in]
            }
            frame 2 {
              n156 = Initialize Array(w630) -> (w629:i32[][])  [unwired: 2 in]
              n157 = Variant To Data(error in=w632, type=w629, Variant=w633) -> (data=w631:i32[][], error out=w636:errorcluster)
              n158 = Flatten To JSON(anything=w631, error in (no error)=w636) -> (JSON string=w635:string, 11:w634:errorcluster)  [unwired: 1 in]
            }
            frame 3 {
              n159 = Initialize Array(w638) -> (w637:i32[][][])  [unwired: 3 in]
              n160 = Variant To Data(error in=w640, type=w637, Variant=w641) -> (data=w639:i32[][][], error out=w644:errorcluster)
              n161 = Flatten To JSON(anything=w639, error in (no error)=w644) -> (JSON string=w643:string, 11:w642:errorcluster)  [unwired: 1 in]
            }
            frame 4 {
              n162 = Initialize Array(w646) -> (w645:i32[][][][])  [unwired: 4 in]
              n163 = Variant To Data(error in=w648, type=w645, Variant=w649) -> (data=w647:i32[][][][], error out=w652:errorcluster)
              n164 = Flatten To JSON(anything=w647, error in (no error)=w652) -> (JSON string=w651:string, 11:w650:errorcluster)  [unwired: 1 in]
            }
          }
        }
        frame "I64" {
          n165 = case shown="1" w654 {
            tunnel: ["" ("JSON string") w667 w675 w683 w691] -> w658
            tunnel: [w660 w666 w674 w682 w690] -> w657
            tunnel: w656 -> [_ w665 w673 w681 w689]
            tunnel: w655 -> [w660 w664 w672 w680 w688]
            tunnel: i64 0 -> [_ w662 w670 w678 w686]
            frame 0, Default {
            }
            frame 1 {
              n166 = Initialize Array(w662) -> (w661:i64[])  [unwired: 1 in]
              n167 = Variant To Data(error in=w664, type=w661, Variant=w665) -> (data=w663:i64[], error out=w668:errorcluster)
              n168 = Flatten To JSON(anything=w663, error in (no error)=w668) -> (JSON string=w667:string, 11:w666:errorcluster)  [unwired: 1 in]
            }
            frame 2 {
              n169 = Initialize Array(w670) -> (w669:i64[][])  [unwired: 2 in]
              n170 = Variant To Data(error in=w672, type=w669, Variant=w673) -> (data=w671:i64[][], error out=w676:errorcluster)
              n171 = Flatten To JSON(anything=w671, error in (no error)=w676) -> (JSON string=w675:string, 11:w674:errorcluster)  [unwired: 1 in]
            }
            frame 3 {
              n172 = Initialize Array(w678) -> (w677:i64[][][])  [unwired: 3 in]
              n173 = Variant To Data(error in=w680, type=w677, Variant=w681) -> (data=w679:i64[][][], error out=w684:errorcluster)
              n174 = Flatten To JSON(anything=w679, error in (no error)=w684) -> (JSON string=w683:string, 11:w682:errorcluster)  [unwired: 1 in]
            }
            frame 4 {
              n175 = Initialize Array(w686) -> (w685:i64[][][][])  [unwired: 4 in]
              n176 = Variant To Data(error in=w688, type=w685, Variant=w689) -> (data=w687:i64[][][][], error out=w692:errorcluster)
              n177 = Flatten To JSON(anything=w687, error in (no error)=w692) -> (JSON string=w691:string, 11:w690:errorcluster)  [unwired: 1 in]
            }
          }
        }
        frame "U8" {
          n178 = case shown="1" w694 {
            tunnel: ["" ("JSON string") w707 w715 w723 w731] -> w698
            tunnel: [w700 w706 w714 w722 w730] -> w697
            tunnel: w696 -> [_ w705 w713 w721 w729]
            tunnel: w695 -> [w700 w704 w712 w720 w728]
            tunnel: u8 0 -> [_ w702 w710 w718 w726]
            frame 0, Default {
            }
            frame 1 {
              n179 = Initialize Array(w702) -> (w701:u8[])  [unwired: 1 in]
              n180 = Variant To Data(error in=w704, type=w701, Variant=w705) -> (data=w703:u8[], error out=w708:errorcluster)
              n181 = Flatten To JSON(anything=w703, error in (no error)=w708) -> (JSON string=w707:string, 11:w706:errorcluster)  [unwired: 1 in]
            }
            frame 2 {
              n182 = Initialize Array(w710) -> (w709:u8[][])  [unwired: 2 in]
              n183 = Variant To Data(error in=w712, type=w709, Variant=w713) -> (data=w711:u8[][], error out=w716:errorcluster)
              n184 = Flatten To JSON(anything=w711, error in (no error)=w716) -> (JSON string=w715:string, 11:w714:errorcluster)  [unwired: 1 in]
            }
            frame 3 {
              n185 = Initialize Array(w718) -> (w717:u8[][][])  [unwired: 3 in]
              n186 = Variant To Data(error in=w720, type=w717, Variant=w721) -> (data=w719:u8[][][], error out=w724:errorcluster)
              n187 = Flatten To JSON(anything=w719, error in (no error)=w724) -> (JSON string=w723:string, 11:w722:errorcluster)  [unwired: 1 in]
            }
            frame 4 {
              n188 = Initialize Array(w726) -> (w725:u8[][][][])  [unwired: 4 in]
              n189 = Variant To Data(error in=w728, type=w725, Variant=w729) -> (data=w727:u8[][][][], error out=w732:errorcluster)
              n190 = Flatten To JSON(anything=w727, error in (no error)=w732) -> (JSON string=w731:string, 11:w730:errorcluster)  [unwired: 1 in]
            }
          }
        }
        frame "U16" {
          n191 = case shown="1" w734 {
            tunnel: ["" ("JSON string") w747 w755 w763 w771] -> w738
            tunnel: [w740 w746 w754 w762 w770] -> w737
            tunnel: w736 -> [_ w745 w753 w761 w769]
            tunnel: w735 -> [w740 w744 w752 w760 w768]
            tunnel: u16 0 -> [_ w742 w750 w758 w766]
            frame 0, Default {
            }
            frame 1 {
              n192 = Initialize Array(w742) -> (w741:u16[])  [unwired: 1 in]
              n193 = Variant To Data(error in=w744, type=w741, Variant=w745) -> (data=w743:u16[], error out=w748:errorcluster)
              n194 = Flatten To JSON(anything=w743, error in (no error)=w748) -> (JSON string=w747:string, 11:w746:errorcluster)  [unwired: 1 in]
            }
            frame 2 {
              n195 = Initialize Array(w750) -> (w749:u16[][])  [unwired: 2 in]
              n196 = Variant To Data(error in=w752, type=w749, Variant=w753) -> (data=w751:u16[][], error out=w756:errorcluster)
              n197 = Flatten To JSON(anything=w751, error in (no error)=w756) -> (JSON string=w755:string, 11:w754:errorcluster)  [unwired: 1 in]
            }
            frame 3 {
              n198 = Initialize Array(w758) -> (w757:u16[][][])  [unwired: 3 in]
              n199 = Variant To Data(error in=w760, type=w757, Variant=w761) -> (data=w759:u16[][][], error out=w764:errorcluster)
              n200 = Flatten To JSON(anything=w759, error in (no error)=w764) -> (JSON string=w763:string, 11:w762:errorcluster)  [unwired: 1 in]
            }
            frame 4 {
              n201 = Initialize Array(w766) -> (w765:u16[][][][])  [unwired: 4 in]
              n202 = Variant To Data(error in=w768, type=w765, Variant=w769) -> (data=w767:u16[][][][], error out=w772:errorcluster)
              n203 = Flatten To JSON(anything=w767, error in (no error)=w772) -> (JSON string=w771:string, 11:w770:errorcluster)  [unwired: 1 in]
            }
          }
        }
        frame "U32" {
          n204 = case shown="1" w774 {
            tunnel: ["" ("JSON string") w787 w795 w803 w811] -> w778
            tunnel: [w780 w786 w794 w802 w810] -> w777
            tunnel: w776 -> [_ w785 w793 w801 w809]
            tunnel: w775 -> [w780 w784 w792 w800 w808]
            tunnel: u32 0 -> [_ w782 w790 w798 w806]
            frame 0, Default {
            }
            frame 1 {
              n205 = Initialize Array(w782) -> (w781:u32[])  [unwired: 1 in]
              n206 = Variant To Data(error in=w784, type=w781, Variant=w785) -> (data=w783:u32[], error out=w788:errorcluster)
              n207 = Flatten To JSON(anything=w783, error in (no error)=w788) -> (JSON string=w787:string, 11:w786:errorcluster)  [unwired: 1 in]
            }
            frame 2 {
              n208 = Initialize Array(w790) -> (w789:u32[][])  [unwired: 2 in]
              n209 = Variant To Data(error in=w792, type=w789, Variant=w793) -> (data=w791:u32[][], error out=w796:errorcluster)
              n210 = Flatten To JSON(anything=w791, error in (no error)=w796) -> (JSON string=w795:string, 11:w794:errorcluster)  [unwired: 1 in]
            }
            frame 3 {
              n211 = Initialize Array(w798) -> (w797:u32[][][])  [unwired: 3 in]
              n212 = Variant To Data(error in=w800, type=w797, Variant=w801) -> (data=w799:u32[][][], error out=w804:errorcluster)
              n213 = Flatten To JSON(anything=w799, error in (no error)=w804) -> (JSON string=w803:string, 11:w802:errorcluster)  [unwired: 1 in]
            }
            frame 4 {
              n214 = Initialize Array(w806) -> (w805:u32[][][][])  [unwired: 4 in]
              n215 = Variant To Data(error in=w808, type=w805, Variant=w809) -> (data=w807:u32[][][][], error out=w812:errorcluster)
              n216 = Flatten To JSON(anything=w807, error in (no error)=w812) -> (JSON string=w811:string, 11:w810:errorcluster)  [unwired: 1 in]
            }
          }
        }
        frame "U64" {
          n217 = case shown="1" w814 {
            tunnel: ["" ("JSON string") w827 w835 w843 w851] -> w818
            tunnel: [w820 w826 w834 w842 w850] -> w817
            tunnel: w816 -> [_ w825 w833 w841 w849]
            tunnel: w815 -> [w820 w824 w832 w840 w848]
            tunnel: u64 0 -> [_ w822 w830 w838 w846]
            frame 0, Default {
            }
            frame 1 {
              n218 = Initialize Array(w822) -> (w821:u64[])  [unwired: 1 in]
              n219 = Variant To Data(error in=w824, type=w821, Variant=w825) -> (data=w823:u64[], error out=w828:errorcluster)
              n220 = Flatten To JSON(anything=w823, error in (no error)=w828) -> (JSON string=w827:string, 11:w826:errorcluster)  [unwired: 1 in]
            }
            frame 2 {
              n221 = Initialize Array(w830) -> (w829:u64[][])  [unwired: 2 in]
              n222 = Variant To Data(error in=w832, type=w829, Variant=w833) -> (data=w831:u64[][], error out=w836:errorcluster)
              n223 = Flatten To JSON(anything=w831, error in (no error)=w836) -> (JSON string=w835:string, 11:w834:errorcluster)  [unwired: 1 in]
            }
            frame 3 {
              n224 = Initialize Array(w838) -> (w837:u64[][][])  [unwired: 3 in]
              n225 = Variant To Data(error in=w840, type=w837, Variant=w841) -> (data=w839:u64[][][], error out=w844:errorcluster)
              n226 = Flatten To JSON(anything=w839, error in (no error)=w844) -> (JSON string=w843:string, 11:w842:errorcluster)  [unwired: 1 in]
            }
            frame 4 {
              n227 = Initialize Array(w846) -> (w845:u64[][][][])  [unwired: 4 in]
              n228 = Variant To Data(error in=w848, type=w845, Variant=w849) -> (data=w847:u64[][][][], error out=w852:errorcluster)
              n229 = Flatten To JSON(anything=w847, error in (no error)=w852) -> (JSON string=w851:string, 11:w850:errorcluster)  [unwired: 1 in]
            }
          }
        }
        frame "Single Float" {
          n230 = case shown="1" w854 {
            tunnel: ["" ("JSON string") w867 w875 w883 w891] -> w858
            tunnel: [w860 w866 w874 w882 w890] -> w857
            tunnel: w856 -> [_ w865 w873 w881 w889]
            tunnel: w855 -> [w860 w864 w872 w880 w888]
            tunnel: sgl 0.0 -> [_ w862 w870 w878 w886]
            frame 0, Default {
            }
            frame 1 {
              n231 = Initialize Array(w862) -> (w861:sgl[])  [unwired: 1 in]
              n232 = Variant To Data(error in=w864, type=w861, Variant=w865) -> (data=w863:sgl[], error out=w868:errorcluster)
              n233 = Flatten To JSON(anything=w863, error in (no error)=w868) -> (JSON string=w867:string, 11:w866:errorcluster)  [unwired: 1 in]
            }
            frame 2 {
              n234 = Initialize Array(w870) -> (w869:sgl[][])  [unwired: 2 in]
              n235 = Variant To Data(error in=w872, type=w869, Variant=w873) -> (data=w871:sgl[][], error out=w876:errorcluster)
              n236 = Flatten To JSON(anything=w871, error in (no error)=w876) -> (JSON string=w875:string, 11:w874:errorcluster)  [unwired: 1 in]
            }
            frame 3 {
              n237 = Initialize Array(w878) -> (w877:sgl[][][])  [unwired: 3 in]
              n238 = Variant To Data(error in=w880, type=w877, Variant=w881) -> (data=w879:sgl[][][], error out=w884:errorcluster)
              n239 = Flatten To JSON(anything=w879, error in (no error)=w884) -> (JSON string=w883:string, 11:w882:errorcluster)  [unwired: 1 in]
            }
            frame 4 {
              n240 = Initialize Array(w886) -> (w885:sgl[][][][])  [unwired: 4 in]
              n241 = Variant To Data(error in=w888, type=w885, Variant=w889) -> (data=w887:sgl[][][][], error out=w892:errorcluster)
              n242 = Flatten To JSON(anything=w887, error in (no error)=w892) -> (JSON string=w891:string, 11:w890:errorcluster)  [unwired: 1 in]
            }
          }
        }
        frame "Double Float" {
          n243 = case shown="1" w894 {
            tunnel: ["" ("JSON string") w907 w915 w923 w931] -> w898
            tunnel: [w900 w906 w914 w922 w930] -> w897
            tunnel: w896 -> [_ w905 w913 w921 w929]
            tunnel: w895 -> [w900 w904 w912 w920 w928]
            tunnel: 0.0 -> [_ w902 w910 w918 w926]
            frame 0, Default {
            }
            frame 1 {
              n244 = Initialize Array(w902) -> (w901:dbl[])  [unwired: 1 in]
              n245 = Variant To Data(error in=w904, type=w901, Variant=w905) -> (data=w903:dbl[], error out=w908:errorcluster)
              n246 = Flatten To JSON(anything=w903, error in (no error)=w908) -> (JSON string=w907:string, 11:w906:errorcluster)  [unwired: 1 in]
            }
            frame 2 {
              n247 = Initialize Array(w910) -> (w909:dbl[][])  [unwired: 2 in]
              n248 = Variant To Data(error in=w912, type=w909, Variant=w913) -> (data=w911:dbl[][], error out=w916:errorcluster)
              n249 = Flatten To JSON(anything=w911, error in (no error)=w916) -> (JSON string=w915:string, 11:w914:errorcluster)  [unwired: 1 in]
            }
            frame 3 {
              n250 = Initialize Array(w918) -> (w917:dbl[][][])  [unwired: 3 in]
              n251 = Variant To Data(error in=w920, type=w917, Variant=w921) -> (data=w919:dbl[][][], error out=w924:errorcluster)
              n252 = Flatten To JSON(anything=w919, error in (no error)=w924) -> (JSON string=w923:string, 11:w922:errorcluster)  [unwired: 1 in]
            }
            frame 4 {
              n253 = Initialize Array(w926) -> (w925:dbl[][][][])  [unwired: 4 in]
              n254 = Variant To Data(error in=w928, type=w925, Variant=w929) -> (data=w927:dbl[][][][], error out=w932:errorcluster)
              n255 = Flatten To JSON(anything=w927, error in (no error)=w932) -> (JSON string=w931:string, 11:w930:errorcluster)  [unwired: 1 in]
            }
          }
        }
        frame "Extended Float" {
          n256 = case shown="1" w934 {
            tunnel: ["" ("JSON string") w947 w955 w963 w971] -> w938
            tunnel: [w940 w946 w954 w962 w970] -> w937
            tunnel: w936 -> [_ w945 w953 w961 w969]
            tunnel: w935 -> [w940 w944 w952 w960 w968]
            tunnel: ext 0.0 -> [_ w942 w950 w958 w966]
            frame 0, Default {
            }
            frame 1 {
              n257 = Initialize Array(w942) -> (w941:ext[])  [unwired: 1 in]
              n258 = Variant To Data(error in=w944, type=w941, Variant=w945) -> (data=w943:ext[], error out=w948:errorcluster)
              n259 = Flatten To JSON(anything=w943, error in (no error)=w948) -> (JSON string=w947:string, 11:w946:errorcluster)  [unwired: 1 in]
            }
            frame 2 {
              n260 = Initialize Array(w950) -> (w949:ext[][])  [unwired: 2 in]
              n261 = Variant To Data(error in=w952, type=w949, Variant=w953) -> (data=w951:ext[][], error out=w956:errorcluster)
              n262 = Flatten To JSON(anything=w951, error in (no error)=w956) -> (JSON string=w955:string, 11:w954:errorcluster)  [unwired: 1 in]
            }
            frame 3 {
              n263 = Initialize Array(w958) -> (w957:ext[][][])  [unwired: 3 in]
              n264 = Variant To Data(error in=w960, type=w957, Variant=w961) -> (data=w959:ext[][][], error out=w964:errorcluster)
              n265 = Flatten To JSON(anything=w959, error in (no error)=w964) -> (JSON string=w963:string, 11:w962:errorcluster)  [unwired: 1 in]
            }
            frame 4 {
              n266 = Initialize Array(w966) -> (w965:ext[][][][])  [unwired: 4 in]
              n267 = Variant To Data(error in=w968, type=w965, Variant=w969) -> (data=w967:ext[][][][], error out=w972:errorcluster)
              n268 = Flatten To JSON(anything=w967, error in (no error)=w972) -> (JSON string=w971:string, 11:w970:errorcluster)  [unwired: 1 in]
            }
          }
        }
        frame "Single Float With Unit" {
          n269 = case shown="1" w974 {
            tunnel: ["" ("JSON string") w987 w995 w1003 w1011] -> w978
            tunnel: [w980 w986 w994 w1002 w1010] -> w977
            tunnel: w976 -> [_ w985 w993 w1001 w1009]
            tunnel: w975 -> [w980 w984 w992 w1000 w1008]
            tunnel: sgl 0.0 -> [_ w982 w990 w998 w1006]
            frame 0, Default {
            }
            frame 1 {
              n270 = Initialize Array(w982) -> (w981:sgl[])  [unwired: 1 in]
              n271 = Variant To Data(error in=w984, type=w981, Variant=w985) -> (data=w983:sgl[], error out=w988:errorcluster)
              n272 = Flatten To JSON(anything=w983, error in (no error)=w988) -> (JSON string=w987:string, 11:w986:errorcluster)  [unwired: 1 in]
            }
            frame 2 {
              n273 = Initialize Array(w990) -> (w989:sgl[][])  [unwired: 2 in]
              n274 = Variant To Data(error in=w992, type=w989, Variant=w993) -> (data=w991:sgl[][], error out=w996:errorcluster)
              n275 = Flatten To JSON(anything=w991, error in (no error)=w996) -> (JSON string=w995:string, 11:w994:errorcluster)  [unwired: 1 in]
            }
            frame 3 {
              n276 = Initialize Array(w998) -> (w997:sgl[][][])  [unwired: 3 in]
              n277 = Variant To Data(error in=w1000, type=w997, Variant=w1001) -> (data=w999:sgl[][][], error out=w1004:errorcluster)
              n278 = Flatten To JSON(anything=w999, error in (no error)=w1004) -> (JSON string=w1003:string, 11:w1002:errorcluster)  [unwired: 1 in]
            }
            frame 4 {
              n279 = Initialize Array(w1006) -> (w1005:sgl[][][][])  [unwired: 4 in]
              n280 = Variant To Data(error in=w1008, type=w1005, Variant=w1009) -> (data=w1007:sgl[][][][], error out=w1012:errorcluster)
              n281 = Flatten To JSON(anything=w1007, error in (no error)=w1012) -> (JSON string=w1011:string, 11:w1010:errorcluster)  [unwired: 1 in]
            }
          }
        }
        frame "Double Float With Unit" {
          n282 = case shown="1" w1014 {
            tunnel: ["" ("JSON string") w1027 w1035 w1043 w1051] -> w1018
            tunnel: [w1020 w1026 w1034 w1042 w1050] -> w1017
            tunnel: w1016 -> [_ w1025 w1033 w1041 w1049]
            tunnel: w1015 -> [w1020 w1024 w1032 w1040 w1048]
            tunnel: 0.0 -> [_ w1022 w1030 w1038 w1046]
            frame 0, Default {
            }
            frame 1 {
              n283 = Initialize Array(w1022) -> (w1021:dbl[])  [unwired: 1 in]
              n284 = Variant To Data(error in=w1024, type=w1021, Variant=w1025) -> (data=w1023:dbl[], error out=w1028:errorcluster)
              n285 = Flatten To JSON(anything=w1023, error in (no error)=w1028) -> (JSON string=w1027:string, 11:w1026:errorcluster)  [unwired: 1 in]
            }
            frame 2 {
              n286 = Initialize Array(w1030) -> (w1029:dbl[][])  [unwired: 2 in]
              n287 = Variant To Data(error in=w1032, type=w1029, Variant=w1033) -> (data=w1031:dbl[][], error out=w1036:errorcluster)
              n288 = Flatten To JSON(anything=w1031, error in (no error)=w1036) -> (JSON string=w1035:string, 11:w1034:errorcluster)  [unwired: 1 in]
            }
            frame 3 {
              n289 = Initialize Array(w1038) -> (w1037:dbl[][][])  [unwired: 3 in]
              n290 = Variant To Data(error in=w1040, type=w1037, Variant=w1041) -> (data=w1039:dbl[][][], error out=w1044:errorcluster)
              n291 = Flatten To JSON(anything=w1039, error in (no error)=w1044) -> (JSON string=w1043:string, 11:w1042:errorcluster)  [unwired: 1 in]
            }
            frame 4 {
              n292 = Initialize Array(w1046) -> (w1045:dbl[][][][])  [unwired: 4 in]
              n293 = Variant To Data(error in=w1048, type=w1045, Variant=w1049) -> (data=w1047:dbl[][][][], error out=w1052:errorcluster)
              n294 = Flatten To JSON(anything=w1047, error in (no error)=w1052) -> (JSON string=w1051:string, 11:w1050:errorcluster)  [unwired: 1 in]
            }
          }
        }
        frame "Extended Float With Unit" {
          n295 = case shown="1" w1054 {
            tunnel: ["" ("JSON string") w1067 w1075 w1083 w1091] -> w1058
            tunnel: [w1060 w1066 w1074 w1082 w1090] -> w1057
            tunnel: w1056 -> [_ w1065 w1073 w1081 w1089]
            tunnel: w1055 -> [w1060 w1064 w1072 w1080 w1088]
            tunnel: ext 0.0 -> [_ w1062 w1070 w1078 w1086]
            frame 0, Default {
            }
            frame 1 {
              n296 = Initialize Array(w1062) -> (w1061:ext[])  [unwired: 1 in]
              n297 = Variant To Data(error in=w1064, type=w1061, Variant=w1065) -> (data=w1063:ext[], error out=w1068:errorcluster)
              n298 = Flatten To JSON(anything=w1063, error in (no error)=w1068) -> (JSON string=w1067:string, 11:w1066:errorcluster)  [unwired: 1 in]
            }
            frame 2 {
              n299 = Initialize Array(w1070) -> (w1069:ext[][])  [unwired: 2 in]
              n300 = Variant To Data(error in=w1072, type=w1069, Variant=w1073) -> (data=w1071:ext[][], error out=w1076:errorcluster)
              n301 = Flatten To JSON(anything=w1071, error in (no error)=w1076) -> (JSON string=w1075:string, 11:w1074:errorcluster)  [unwired: 1 in]
            }
            frame 3 {
              n302 = Initialize Array(w1078) -> (w1077:ext[][][])  [unwired: 3 in]
              n303 = Variant To Data(error in=w1080, type=w1077, Variant=w1081) -> (data=w1079:ext[][][], error out=w1084:errorcluster)
              n304 = Flatten To JSON(anything=w1079, error in (no error)=w1084) -> (JSON string=w1083:string, 11:w1082:errorcluster)  [unwired: 1 in]
            }
            frame 4 {
              n305 = Initialize Array(w1086) -> (w1085:ext[][][][])  [unwired: 4 in]
              n306 = Variant To Data(error in=w1088, type=w1085, Variant=w1089) -> (data=w1087:ext[][][][], error out=w1092:errorcluster)
              n307 = Flatten To JSON(anything=w1087, error in (no error)=w1092) -> (JSON string=w1091:string, 11:w1090:errorcluster)  [unwired: 1 in]
            }
          }
        }
        frame "Boolean" {
          n308 = case shown="1" w1094 {
            tunnel: ["" ("JSON string") w1107 w1115 w1123 w1131] -> w1098
            tunnel: [w1100 w1106 w1114 w1122 w1130] -> w1097
            tunnel: w1096 -> [_ w1105 w1113 w1121 w1129]
            tunnel: w1095 -> [w1100 w1104 w1112 w1120 w1128]
            tunnel: FALSE -> [_ w1102 w1110 w1118 w1126]
            frame 0, Default {
            }
            frame 1 {
              n309 = Initialize Array(w1102) -> (w1101:bool[])  [unwired: 1 in]
              n310 = Variant To Data(error in=w1104, type=w1101, Variant=w1105) -> (data=w1103:bool[], error out=w1108:errorcluster)
              n311 = Flatten To JSON(anything=w1103, error in (no error)=w1108) -> (JSON string=w1107:string, 11:w1106:errorcluster)  [unwired: 1 in]
            }
            frame 2 {
              n312 = Initialize Array(w1110) -> (w1109:bool[][])  [unwired: 2 in]
              n313 = Variant To Data(error in=w1112, type=w1109, Variant=w1113) -> (data=w1111:bool[][], error out=w1116:errorcluster)
              n314 = Flatten To JSON(anything=w1111, error in (no error)=w1116) -> (JSON string=w1115:string, 11:w1114:errorcluster)  [unwired: 1 in]
            }
            frame 3 {
              n315 = Initialize Array(w1118) -> (w1117:bool[][][])  [unwired: 3 in]
              n316 = Variant To Data(error in=w1120, type=w1117, Variant=w1121) -> (data=w1119:bool[][][], error out=w1124:errorcluster)
              n317 = Flatten To JSON(anything=w1119, error in (no error)=w1124) -> (JSON string=w1123:string, 11:w1122:errorcluster)  [unwired: 1 in]
            }
            frame 4 {
              n318 = Initialize Array(w1126) -> (w1125:bool[][][][])  [unwired: 4 in]
              n319 = Variant To Data(error in=w1128, type=w1125, Variant=w1129) -> (data=w1127:bool[][][][], error out=w1132:errorcluster)
              n320 = Flatten To JSON(anything=w1127, error in (no error)=w1132) -> (JSON string=w1131:string, 11:w1130:errorcluster)  [unwired: 1 in]
            }
          }
        }
        frame "String" {
          n321 = case shown="1" w1134 {
            tunnel: ["" ("JSON string") w1147 w1155 w1163 w1171] -> w1138
            tunnel: [w1140 w1146 w1154 w1162 w1170] -> w1137
            tunnel: w1136 -> [_ w1145 w1153 w1161 w1169]
            tunnel: w1135 -> [w1140 w1144 w1152 w1160 w1168]
            tunnel: "" -> [_ w1142 w1150 w1158 w1166]
            frame 0, Default {
            }
            frame 1 {
              n322 = Initialize Array(w1142) -> (w1141:string[])  [unwired: 1 in]
              n323 = Variant To Data(error in=w1144, type=w1141, Variant=w1145) -> (data=w1143:string[], error out=w1148:errorcluster)
              n324 = Flatten To JSON(anything=w1143, error in (no error)=w1148) -> (JSON string=w1147:string, 11:w1146:errorcluster)  [unwired: 1 in]
            }
            frame 2 {
              n325 = Initialize Array(w1150) -> (w1149:string[][])  [unwired: 2 in]
              n326 = Variant To Data(error in=w1152, type=w1149, Variant=w1153) -> (data=w1151:string[][], error out=w1156:errorcluster)
              n327 = Flatten To JSON(anything=w1151, error in (no error)=w1156) -> (JSON string=w1155:string, 11:w1154:errorcluster)  [unwired: 1 in]
            }
            frame 3 {
              n328 = Initialize Array(w1158) -> (w1157:string[][][])  [unwired: 3 in]
              n329 = Variant To Data(error in=w1160, type=w1157, Variant=w1161) -> (data=w1159:string[][][], error out=w1164:errorcluster)
              n330 = Flatten To JSON(anything=w1159, error in (no error)=w1164) -> (JSON string=w1163:string, 11:w1162:errorcluster)  [unwired: 1 in]
            }
            frame 4 {
              n331 = Initialize Array(w1166) -> (w1165:string[][][][])  [unwired: 4 in]
              n332 = Variant To Data(error in=w1168, type=w1165, Variant=w1169) -> (data=w1167:string[][][][], error out=w1172:errorcluster)
              n333 = Flatten To JSON(anything=w1167, error in (no error)=w1172) -> (JSON string=w1171:string, 11:w1170:errorcluster)  [unwired: 1 in]
            }
          }
        }
        frame "Path" {
          n334 = case shown="1" w1174 {
            tunnel: ["" ("JSON string") w1190] -> w1178
            tunnel: [w1180 w1189] -> w1177
            tunnel: w1176 -> [_ w1188]
            tunnel: w1175 -> [w1180 w1187]
            tunnel: path "" -> [_ w1186]
            frame 0, Default {
            }
            frame 1 {
              n335 = Initialize Array(w1186) -> (w1185:path[])  [unwired: 1 in]
              n336 = Variant To Data(error in=w1187, type=w1185, Variant=w1188) -> (data=w1184:path[], error out=w1183:errorcluster)
              n337 = for {
                tunnel: w1184 -> [w1193] mode=indexing
                shift-right: [w1192] -> w1182
                shift-left: w1183 -> [w1192]
                tunnel: [w1191] -> w1181 mode=indexing
                n338 = Path To String(path=w1193) -> (string=w1191:string)
              }
              n339 = Flatten To JSON(anything=w1181, error in (no error)=w1182) -> (JSON string=w1190:string, 11:w1189:errorcluster)  [unwired: 1 in]
            }
          }
        }
        frame "Picture" {
          n340 = call "Empty Picture"() -> ("empty picture"=w1194:picture)
          n341 = case shown="1" w1195 {
            tunnel: ["" ("JSON string") w1202] -> w1199
            tunnel: [w1201 w1204] -> w1198
            tunnel: w1197 -> [_ w1212]
            tunnel: w1196 -> [w1201 w1211]
            tunnel: w1194 -> [_ w1210]
            frame 0, Default {
            }
            frame 1 {
              n342 = Initialize Array(w1210) -> (w1209:picture[])  [unwired: 1 in]
              n343 = Variant To Data(error in=w1211, type=w1209, Variant=w1212) -> (data=w1207:picture[], error out=w1208:errorcluster)
              n344 = for {
                shift-right: [w1215] -> w1204
                shift-left: w1208 -> [w1216]
                tunnel: w1207 -> [w1214] mode=indexing
                tunnel: [w1213] -> w1205 mode=indexing
                n345 = call <vilib>:"Picture to Pixmap.vi"("picture"=w1214) -> ("image data"=w1217:T6)  [unwired: 9 in, 1 out]
                n346 = call <vilib>:"LV Image to PNG Data.vi"("error in (no error)"=w1216, "image data"=w1217) -> ("error out"=w1215:errorcluster, "png data"=w1213:string)  [unwired: 8 in]
              }
              n347 = Array To Spreadsheet String(delimiter (Tab)=",", array=w1205, 3:"%s" ("delimiter (Tab)")) -> (spreadsheet string=w1202:string)
            }
          }
        }
        frame "Enum U8" {
          n348 = case shown="1" w1220 {
            tunnel: ["" ("JSON string") w1227] -> w1224
            tunnel: [w1225 w1230] -> w1223
            tunnel: w1222 -> [_ w1233]
            tunnel: w1221 -> [_ w1235]
            tunnel: u8 0 -> [_ w1238]
            tunnel: w1218 -> [w1225 _]
            frame 0, Default {
            }
            frame 1 {
              n349 = Initialize Array(w1238) -> (w1234:u8[])  [unwired: 1 in]
              n350 = Variant To Data(error in=w1235, type=w1234, Variant=w1233) -> (data=w1232:u8[], error out=w1237:errorcluster)
              n351 = call <vilib>:"Get Numeric Information.vi"("error in (no error)"=w1237, "variant"=w1233) -> ("error out"=w1230:errorcluster, "enum names"=w1236:string[])  [unwired: 6 in, 2 out]
              n352 = for {
                tunnel: w1236 -> [w1241]
                tunnel: w1232 -> [w1240] mode=indexing
                tunnel: [w1239] -> w1231 mode=indexing
                n353 = Index Array(array=w1241, index=w1240) -> (element=w1239:string)
              }
              n354 = Array To Spreadsheet String(delimiter (Tab)=",", array=w1231, 3:"%s" ("delimiter (Tab)")) -> (spreadsheet string=w1227:string)
            }
          }
        }
        frame "Enum U16" {
          n355 = case shown="1" w1244 {
            tunnel: ["" ("JSON string") w1251] -> w1248
            tunnel: [w1249 w1254] -> w1247
            tunnel: w1246 -> [_ w1257]
            tunnel: w1245 -> [_ w1259]
            tunnel: u16 0 -> [_ w1262]
            tunnel: w1242 -> [w1249 _]
            frame 0, Default {
            }
            frame 1 {
              n356 = Initialize Array(w1262) -> (w1258:u16[])  [unwired: 1 in]
              n357 = Variant To Data(error in=w1259, type=w1258, Variant=w1257) -> (data=w1256:u16[], error out=w1261:errorcluster)
              n358 = call <vilib>:"Get Numeric Information.vi"("error in (no error)"=w1261, "variant"=w1257) -> ("error out"=w1254:errorcluster, "enum names"=w1260:string[])  [unwired: 6 in, 2 out]
              n359 = for {
                tunnel: w1260 -> [w1265]
                tunnel: w1256 -> [w1264] mode=indexing
                tunnel: [w1263] -> w1255 mode=indexing
                n360 = Index Array(array=w1265, index=w1264) -> (element=w1263:string)
              }
              n361 = Array To Spreadsheet String(delimiter (Tab)=",", array=w1255, 3:"%s" ("delimiter (Tab)")) -> (spreadsheet string=w1251:string)
            }
          }
        }
        frame "Enum U32" {
          n362 = case shown="1" w1268 {
            tunnel: ["" ("JSON string") w1275] -> w1272
            tunnel: [w1273 w1278] -> w1271
            tunnel: w1270 -> [_ w1281]
            tunnel: w1269 -> [_ w1283]
            tunnel: u32 0 -> [_ w1286]
            tunnel: w1266 -> [w1273 _]
            frame 0, Default {
            }
            frame 1 {
              n363 = Initialize Array(w1286) -> (w1282:u32[])  [unwired: 1 in]
              n364 = Variant To Data(error in=w1283, type=w1282, Variant=w1281) -> (data=w1280:u32[], error out=w1285:errorcluster)
              n365 = call <vilib>:"Get Numeric Information.vi"("error in (no error)"=w1285, "variant"=w1281) -> ("error out"=w1278:errorcluster, "enum names"=w1284:string[])  [unwired: 6 in, 2 out]
              n366 = for {
                tunnel: w1284 -> [w1289]
                tunnel: w1280 -> [w1288] mode=indexing
                tunnel: [w1287] -> w1279 mode=indexing
                n367 = Index Array(array=w1289, index=w1288) -> (element=w1287:string)
              }
              n368 = Array To Spreadsheet String(delimiter (Tab)=",", array=w1279, 3:"%s" ("delimiter (Tab)")) -> (spreadsheet string=w1275:string)
            }
          }
        }
        frame "Enum U64" {
          n369 = case shown="1" w1292 {
            tunnel: ["[]" ("JSON string") w1299] -> w1296
            tunnel: [w1297 w1302] -> w1295
            tunnel: w1294 -> [_ w1305]
            tunnel: w1293 -> [_ w1307]
            tunnel: u64 0 -> [_ w1310]
            tunnel: w1290 -> [w1297 _]
            frame 0, Default {
            }
            frame 1 {
              n370 = Initialize Array(w1310) -> (w1306:u64[])  [unwired: 1 in]
              n371 = Variant To Data(error in=w1307, type=w1306, Variant=w1305) -> (data=w1304:u64[], error out=w1309:errorcluster)
              n372 = call <vilib>:"Get Numeric Information.vi"("error in (no error)"=w1309, "variant"=w1305) -> ("error out"=w1302:errorcluster, "enum names"=w1308:string[])  [unwired: 6 in, 2 out]
              n373 = for {
                tunnel: w1308 -> [w1313]
                tunnel: w1304 -> [w1312] mode=indexing
                tunnel: [w1311] -> w1303 mode=indexing
                n374 = Index Array(array=w1313, index=w1312) -> (element=w1311:string)
              }
              n375 = Array To Spreadsheet String(delimiter (Tab)=",", array=w1303, 3:"%s" ("delimiter (Tab)")) -> (spreadsheet string=w1299:string)
            }
          }
        }
      }
      n376 = Concatenate Strings("\"", w516, "\":[", w520, "]" ("delimiter (Tab)")) -> (w519:string)
    }
    frame "Cluster" {
      # "#TODO: Make this work"
      n377 = call <vilib>:"Get Cluster Information.vi"("error in (no error)"=w1329, "variant"=w1328) -> ("error out"=w1327:errorcluster, "cluster elements"=w1326:variant[])  [unwired: 8 in]
      n378 = for {
        tunnel: w1326 -> [w1338] mode=indexing
        tunnel: w1325 -> [w1340]
        shift-right: [w1339] -> w1320
        shift-left: w1327 -> [w1341]
        shift-right: [w1336] -> w1318
        shift-left: "application/json" -> [w1337]
        tunnel: [w1333] -> w1322 mode=indexing
        tunnel: w1315 -> [w1331]
        n379 = call "Format Control Data Element.vi"("Unsupported Error"=w1340, "error in (no error)"=w1341, "Content Type in"=w1337, "Data"=w1338) -> ("error out"=w1339:errorcluster, "Content Type out"=w1336:string, "JSON string"=w1335:string)  [unwired: 5 in]
        n380 = Concatenate Strings(w1331, ":" ("string"), "{" ("string"), w1335, "}" ("string")) -> (w1333:string)
      }
      n381 = Array To Spreadsheet String(delimiter (Tab)=",", array=w1322, 3:"%s" ("delimiter (Tab)")) -> (spreadsheet string=w1323:string)
      n382 = Concatenate Strings("{" ("delimiter (Tab)"), w1323, "}" ("delimiter (Tab)")) -> (w1319:string)
    }
    frame "Variant" {
      # "#TODO: Make this work"
      n383 = Get Variant Attribute(Variant=w1346, error in=w1344) -> (names=w1342:string[], values=w1345:variant[], error out=w1343:errorcluster)  [unwired: 2 in, 1 out]
      n384 = for {
        tunnel: w1345 -> [w1366] mode=indexing
        tunnel: w1357 -> [w1368]
        shift-right: [w1367] -> w1352
        shift-left: w1343 -> [w1369]
        shift-right: [w1364] -> w1350
        shift-left: "application/json" -> [w1365]
        tunnel: [w1361] -> w1354 mode=indexing
        tunnel: w1342 -> [w1359] mode=indexing
        n385 = call "Format Control Data Element.vi"("Unsupported Error"=w1368, "error in (no error)"=w1369, "Content Type in"=w1365, "Data"=w1366) -> ("error out"=w1367:errorcluster, "Content Type out"=w1364:string, "JSON string"=w1363:string)  [unwired: 5 in]
        n386 = Concatenate Strings(w1359, ":" ("string"), "{" ("string"), w1363, "}" ("string")) -> (w1361:string)
      }
      n387 = Array To Spreadsheet String(delimiter (Tab)=",", array=w1354, 3:"%s" ("delimiter (Tab)")) -> (spreadsheet string=w1355:string)
      n388 = Concatenate Strings("{" ("delimiter (Tab)"), w1355, "}" ("delimiter (Tab)")) -> (w1351:string)
    }
  }
  "Content Type out" <- w2
  "JSON string" <- w3
  "error out" <- w4
